vi "test_Import Bitfile Scalars_All_Error.vi"(8 "error in (no error)":errorcluster, 11 "TestCase in":refnum<class "FPGA Addon Scripting API Unit Tests.lvclass">) -> (0 "error out":errorcluster, 3 "TestCase out":refnum<class "FPGA Addon Scripting API Unit Tests.lvclass">)   [LabVIEW 2021, in "FPGA Addon Scripting API Unit Tests.lvclass"]
uses:
  FPGA Addon Scripting API Unit Tests.lvclass
  APIs/Scripting API/Public/Bitfile Resources/Import Bitfile Scalars (Instances)/Import Scalars - all.vi
  <vilib>/addons/_JKI Toolkits/VI Tester/TestCase.llb/TestCase.lvclass
  FPGA Addon Test Class/FPGA Addon Test Class.lvclass
  APIs/Scripting API/Scripting API.lvlib
  C:/Program Files/National Instruments/LabVIEW 2021/vi.lib/addons/_JKI Toolkits/VI Tester/TestCase.llb/TestCase.lvclass
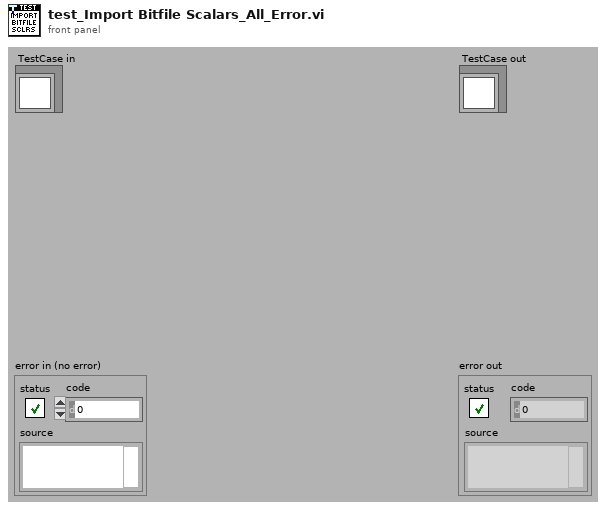
[diagram p1: front panel]
types:
  T1 = typedef "Custom Device API.lvlib/Custom Device Item Ref.ctl" = u64
  T2 = typedef "Scripting API.lvlib/Output Scalar Data.ctl" = cluster{"Bitfile Name":string, "SysDef Channel Name":string, "Imported":bool, "Data Type":T3}
  T3 = typedef "FPGA Addon Shared.lvlib/FPGA Addon Data Type.ctl" = enum8{"<Null>", "I8", "I16", "I32", "I64", "U8", "U16", "U32", "U64", "SGL", "Boolean", "Analog PWM In Settings", "Analog PWM In", "Digital PWM In Settings", "Digital PWM In", "Digital PWM Out", "Sine Out", "FXP", "FXP+/-24.5", "FXP+/-16.5", "FXP+/-32.8", "FXP+/-64.32", "FXP+/-16.7", "FXP+/-20.5", "FXP+/-27.5", "FXP+/-32.16", "FXP+16.3", "FXP+18.3", "Digital Static In", "Digital Static Out", "Digital Static In Settings", "Digital WSS Out", "Quad Encoder Settings", "Quad Encoder In", "Group"}
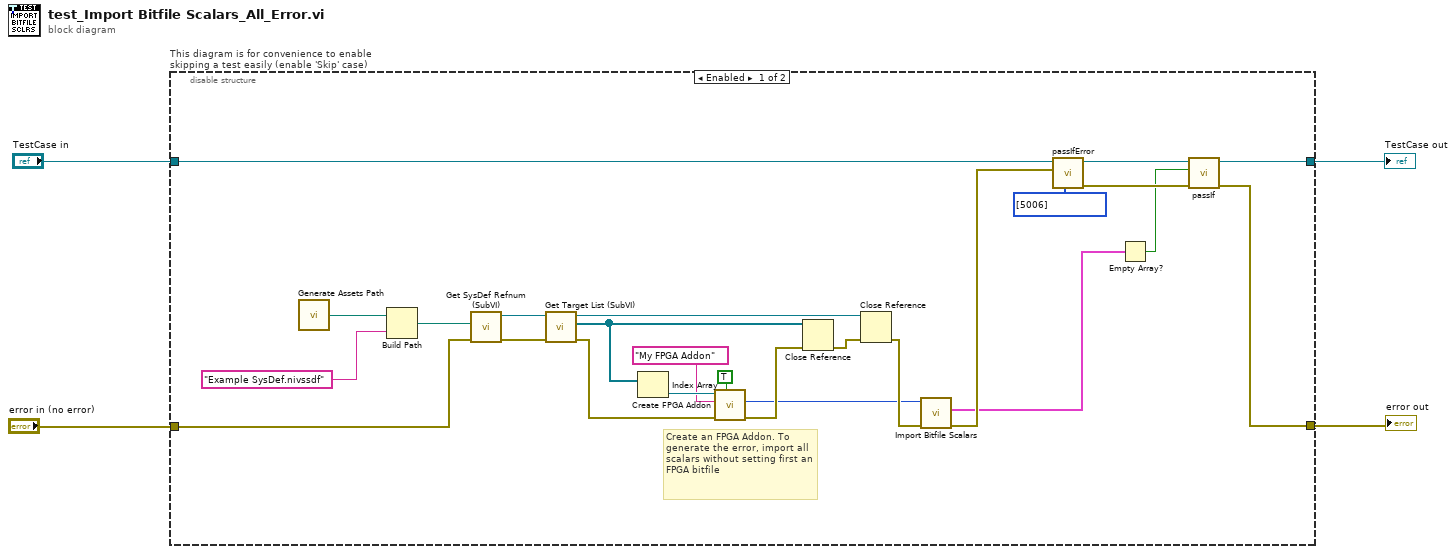
[diagram p0: block diagram]
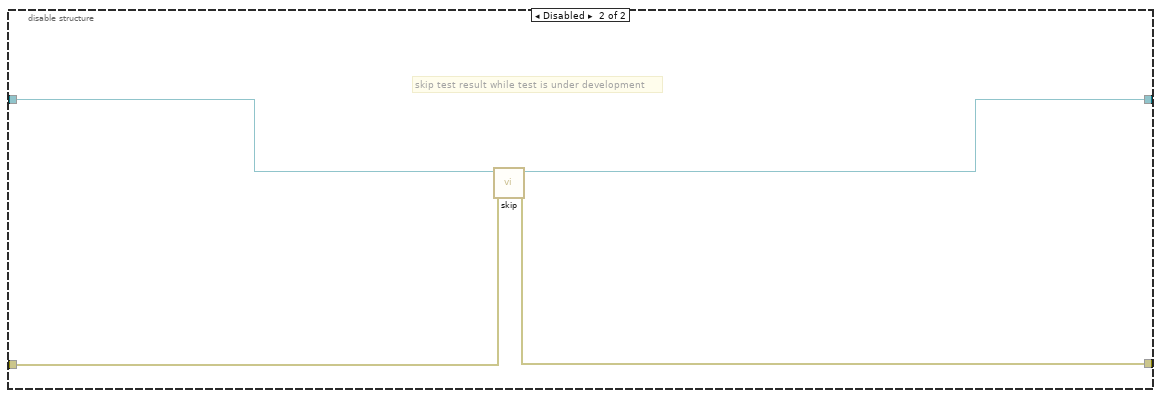
[diagram p2: hidden frame]
diagram:
  n1 = disable-structure "This diagram is for convenience to enable skipping a test easily (enable 'Skip' case)" shown="Enabled" {
    disable-tunnel: "TestCase in" -> [w13 w33]
    disable-tunnel: [w6 w31] -> w1
    disable-tunnel: [w5 w32] -> w3
    disable-tunnel: "error in (no error)" -> [w23 w30]
    frame Enabled {
      # "Create an FPGA Addon. To generate the error, import all scalars without setting first an FPGA bitfile"
      n2 = call "Generate Assets Path.vi"() -> ("Assets path"=w29:path)
      n3 = Build Path(base path=w29, name or relative path="Example SysDef.nivssdf") -> (appended path=w27:path)
      n4 = call "Get SysDef Refnum (SubVI).vi"("error in (no error)"=w23, "System Definition path"=w27) -> ("error out"=w22:errorcluster, "SysDef Refnum out"=w26:refnum<k24>)  [unwired: 8 in]
      n5 = call "Get Target List (SubVI).vi"("error in (no error)"=w22, "SysDef Refnum in"=w26) -> ("error out"=w21:errorcluster, "Target List Refnums"=w20:refnum<k24>[], "SysDef Refnum out"=w19:refnum<k24>)  [unwired: 7 in]
      n6 = Index Array(array=w20) -> (element=w25:refnum<k24>)  [unwired: 1 in]
      n7 = call "Create FPGA Addon.vi"("group scalars"=TRUE, "error in"=w21, "FPGA addon name"="My FPGA Addon", "target in"=w25) -> ("error out"=w17:errorcluster, "FPGA addon refnum"=w14:T1)  [unwired: 5 in, 1 out]
      n8 = Close Reference(reference=w20, error in (no error)=w17) -> (error out=w18:errorcluster)
      n9 = Close Reference(reference=w19, error in (no error)=w18) -> (error out=w15:errorcluster)
      n10 = call-poly "Import Bitfile Scalars.vi"("error in"=w15, "FPGA addon refnum in"=w14) -> ("error out"=w12:errorcluster, "imported bitfile scalars out"=w8:T2[])  [unwired: 7 in, 1 out]
      n11 = call-dynamic "passIfError.vi"("passing error codes (default = any error code)"=i32[] [5006], "error"=w12, "TestCase in"=w13) -> ("error out"=w9:errorcluster, "TestCase out"=w10:refnum<class "FPGA Addon Scripting API Unit Tests.lvclass">)  [unwired: 7 in]
      n12 = Empty Array?(array=w8) -> (empty?=w7:bool)
      n13 = call-dynamic "passIf.vi"("error in (no error)"=w9, "pass"=w7, "TestCase in"=w10) -> ("error out"=w5:errorcluster, "TestCase out"=w6:refnum<class "FPGA Addon Scripting API Unit Tests.lvclass">)  [unwired: 7 in]
    }
    frame Disabled {
      # "skip test result while test is under development"
      n14 = call <vilib>:"skip.vi"("error in (no error)"=w30, "TestCase in"=w33) -> ("error out"=w32:errorcluster, "TestCase out"=w31:refnum<class "FPGA Addon Scripting API Unit Tests.lvclass">)  [unwired: 8 in]
    }
  }
  "error out" <- w3
  "TestCase out" <- w1
